vi "Write Index.vi"(8 "error in (no error)":errorcluster, 10 "Index":cluster{"frame index":i32, "channel index":i32}={"frame index"=0, "channel index"=1} {"channel index" step=1; "frame index" step=1}, 11 "Chroma 190020 in":refnum<class "Chroma 190020.lvclass">) -> (0 "error out":errorcluster, 3 "Chroma 190020 out":refnum<class "Chroma 190020.lvclass">)   [LabVIEW 2025, in "HiPOT.lvlib" / "Chroma 190020.lvclass"]
uses:
  Chroma 190020.lvclass
  Chroma 190020.lvclass/Chroma 190020.ctl
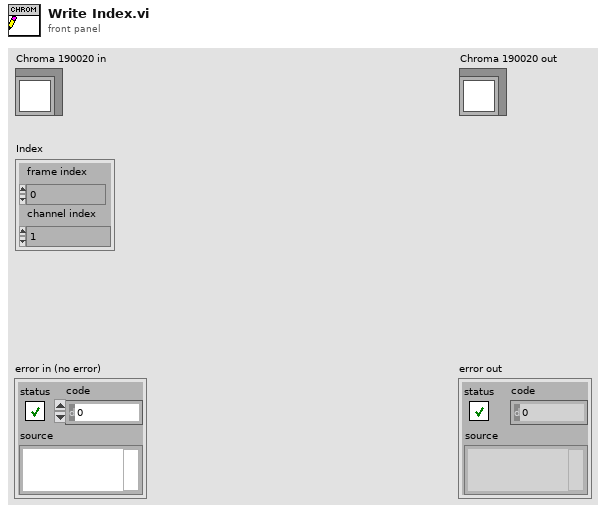
[diagram p1: front panel]
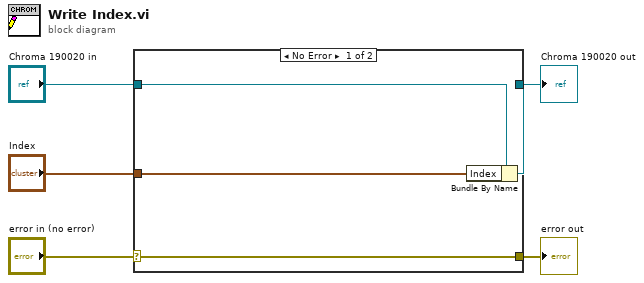
[diagram p0: block diagram]
diagram:
  n1 = case shown="No Error" "error in (no error)" {
    selector: "error in (no error)" -> [w9 w10]
    tunnel: [w9 w10] -> w4
    tunnel: [w7 w11] -> w2
    tunnel: "Chroma 190020 in" -> [w8 w11]
    tunnel: "Index" -> [w6 _]
    frame No Error {
      n2 = Bundle By Name(cluster=w8, "Index"=w6) -> (w7:refnum<class "Chroma 190020.lvclass">)
    }
    frame Error {
    }
  }
  "error out" <- w4
  "Chroma 190020 out" <- w2
